vi "AlliGator Select Parameter Scatter Plot Type.vi"(8 "Error In":errorcluster, 11 "Parameter Names":string[](array[string])) -> (0 "Error Out":errorcluster, 1 "Parameter 2":u16(ring)=3, 2 "Parameter 1":u16(ring)=3, 3 "Cancelled?":bool)   [LabVIEW 2021, in "AlliGator Parameter Map.lvlib"]
doc: "Dialog to select parameter 1 and parameter 2 to be computed for a Phasor Plot of the Phasor Graph."
uses:
  AlliGator Parameter Map.lvlib
panel:
  in  "Cancel":bool
  in  "OK":bool
  in  "Parameter 2":u16(ring)=5
  in  "Parameter 1":u16(ring)=3
  # "Select parameters to export as scatter plot:\n\n- horizontal axis: Parameter 1\n- vertical axis: Parameter 2"
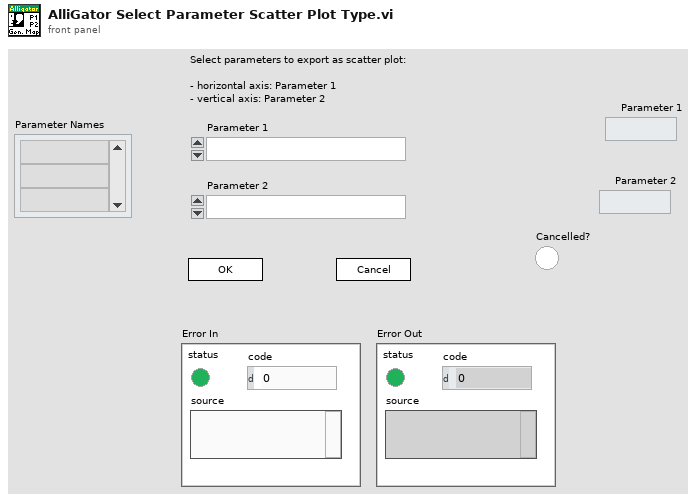
[diagram p1: front panel]
types:
  T1 = enum32{"Invalid", "Standard", "Closed", "Hidden", "Minimized", "Maximized"}
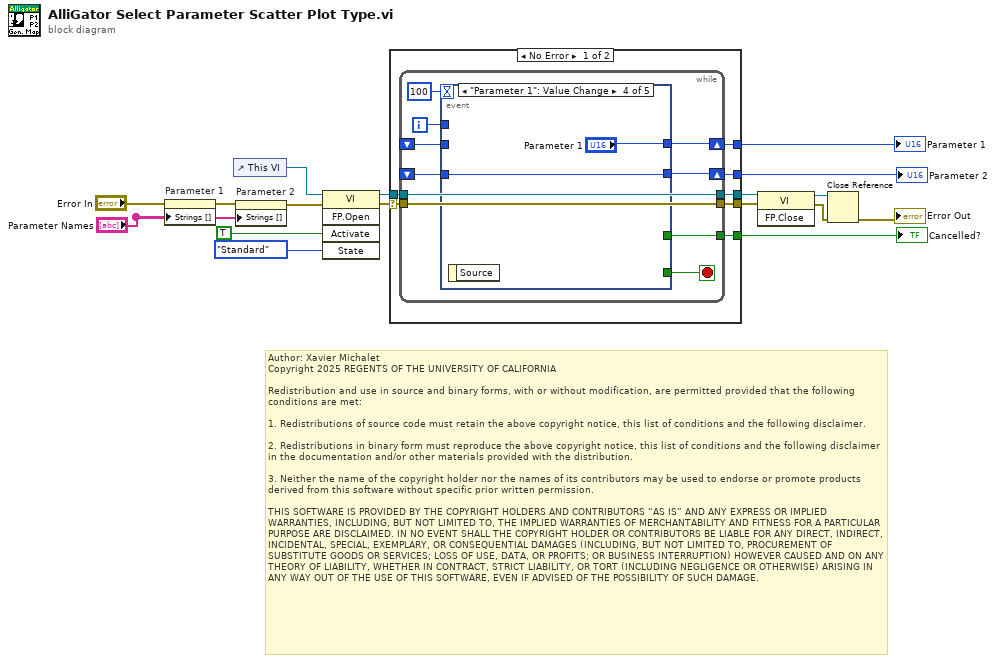
[diagram p0: block diagram]
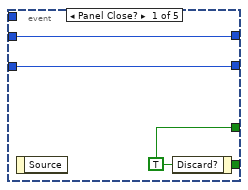
[diagram p2: hidden frame]
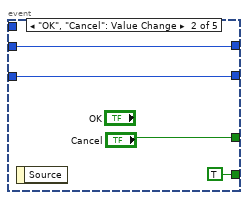
[diagram p3: hidden frame]
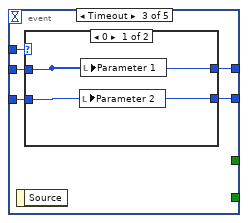
[diagram p4: hidden frame]
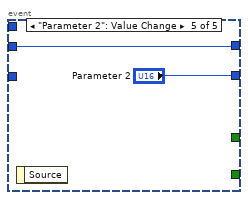
[diagram p6: hidden frame]
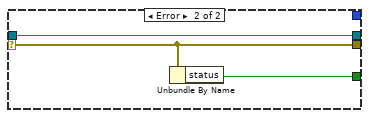
[diagram p7: hidden frame]
diagram:
  # "Author: Xavier Michalet\nCopyright 2025 REGENTS OF THE UNIVERSITY OF CALIFORNIA\n\nRedistribution and use in source and binary forms, with or without modification, are permitted provided that the following conditions are met:\n\n1. Redistributions of source code must retain the above copyright notice, this list of conditions and the following disclaimer.\n\n2. Redistributions in binary form must reproduce the above copyright notice, this list of conditions and the following disclaimer in the documentation and/or other materials provided with the distribution.\n\n3. Neither the name of the copyright holder nor the names of its contributors may be used to endorse or promote products derived from this software without specific prior written permission.\n\nTHIS SOFTWARE IS PROVIDED BY THE COPYRIGHT HOLDERS AND CONTRIBUTORS “AS IS” AND ANY EXPRESS OR IMPLIED WARRANTIES, INCLUDING, BUT NOT LIMITED TO, THE IMPLIED WARRANTIES OF MERCHANTABILITY AND FITNESS FOR A PARTICULAR PURPOSE ARE DISCLAIMED. IN NO EVENT SHALL THE COPYRIGHT HOLDER OR CONTRIBUTORS BE LIABLE FOR ANY DIRECT, INDIRECT, INCIDENTAL, SPECIAL, EXEMPLARY, OR CONSEQUENTIAL DAMAGES (INCLUDING, BUT NOT LIMITED TO, PROCUREMENT OF SUBSTITUTE GOODS OR SERVICES; LOSS OF USE, DATA, OR PROFITS; OR BUSINESS INTERRUPTION) HOWEVER CAUSED AND ON ANY THEORY OF LIABILITY, WHETHER IN CONTRACT, STRICT LIABILITY, OR TORT (INCLUDING NEGLIGENCE OR OTHERWISE) ARISING IN ANY WAY OUT OF THE USE OF THIS SOFTWARE, EVEN IF ADVISED OF THE POSSIBILITY OF SUCH DAMAGE."
  n1 = property on="Parameter 1" class="Ring (strict)"(error in="Error In", "Strings []"="Parameter Names") -> (error out=w3:errorcluster)  [unwired: 1 in, 1 out]
  n2 = control-ref of="This VI"() -> (w13:refnum<vi>)
  n3 = property on="Parameter 2" class="Ring (strict)"(error in=w3, "Strings []"="Parameter Names") -> (error out=w1:errorcluster)  [unwired: 1 in, 1 out]
  n4 = invoke class="VI" method="FP.Open"(reference=w13, error in=w1, "Activate"=TRUE ("Activate?"), "State"=T1."Standard") -> (reference out=w9:refnum<vi>, error out=w10:errorcluster)  [unwired: 1 in, 3 out]
  n5 = case shown="No Error" w10 {
    selector: w10 -> [w21 w56]
    tunnel: [w24 w55] -> w17
    tunnel: [w23 _] -> w16
    tunnel: [w22 _] -> w15
    tunnel: w9 -> [w20 w57]
    tunnel: [w19 w57] -> w8
    tunnel: [w18 w56] -> w7
    frame No Error {
      n6 = while {
        tunnel: [w33] -> w24
        shift-right: [w29] -> w23
        shift-left: _ -> [w30]
        shift-right: [w27] -> w22
        shift-left: _ -> [w28]
        tunnel: w21 -> [w25]
        tunnel: [w26] -> w19
        tunnel: w20 -> [w26]
        tunnel: [w25] -> w18
        i -> [w31]
        stop <- w34 stop-if-true
        n7 = event shown="[3] \"Parameter 1\": Value Change" {
          selector: _ -> [_ _ _ _ _]
          dyn-events: _ -> [_ _ _ _ _]
          timeout: 100 -> [_ _ _ _ _]
          tunnel: [w37 TRUE ("Discard?") _ _ _] -> w34
          tunnel: [w37 "Cancel" _ _ _] -> w33
          tunnel: w31 -> [_ _ w46 _ _]
          tunnel: w30 -> [w36 w39 w45 _ w53]
          tunnel: [w36 w39 w44 "Parameter 1" w53] -> w29
          tunnel: w28 -> [w35 w38 w43 w51 _]
          tunnel: [w35 w38 w42 w51 "Parameter 2"] -> w27
          event Panel Close? {
            w37 = TRUE ("Discard?")
            n8 = event-data() -> ()  [unwired: 1 in, 1 out]
            n9 = event-data("Discard?"=w37) -> ()  [unwired: 1 in, 1 out]
          }
          event "OK", "Cancel": Value Change {
            n10 = event-data() -> ()  [unwired: 1 in, 1 out]
          }
          event Timeout {
            n11 = event-data() -> ()  [unwired: 1 in, 1 out]
            n12 = case shown="0" w46 {
              tunnel: w45 -> [w48 w50]
              tunnel: [w48 w50] -> w44
              tunnel: w43 -> [w47 w49]
              tunnel: [w47 w49] -> w42
              frame 0 {
                n13 = local write "Parameter 2"(w47) -> ()
                n14 = local write "Parameter 1"(w48) -> ()
              }
              frame 1, Default {
              }
            }
          }
          event "Parameter 1": Value Change {
            n15 = event-data() -> ()  [unwired: 1 in, 1 out]
          }
          event "Parameter 2": Value Change {
            n16 = event-data() -> ()  [unwired: 1 in, 1 out]
          }
        }
      }
    }
    frame Error {
      n17 = Unbundle By Name(w56) -> ("status"=w55:bool)
    }
  }
  "Parameter 1" <- w16
  "Parameter 2" <- w15
  "Cancelled?" <- w17
  n18 = invoke class="VI" method="FP.Close"(reference=w8, error in=w7) -> (reference out=w6:refnum<vi>, error out=w5:errorcluster)  [unwired: 1 in, 1 out]
  n19 = Close Reference(reference=w6, error in (no error)=w5) -> (error out=→"Error Out":errorcluster)
